vi "Populate Valid Y Variable Pointer IDs.vi"(8 "error in (no error)":errorcluster, 11 "Conditional Dialog in":refnum<class "Conditional Dialog.lvclass">) -> (0 "error out":errorcluster, 3 "Conditional Dialog out":refnum<class "Conditional Dialog.lvclass">)   [LabVIEW 2017, in "Conditional Dialog.lvclass"]
uses:
  <vilib>/gpm_packages/@cs/Test-executive-builder/Source/Test Executive Builder Dialogs/Edit Conditional Dialog/Conditional Dialog.lvclass
  <vilib>/gpm_packages/@cs/Test-executive-builder/Source/Test Executive Builder Dialogs/Edit Conditional Dialog/Conditional Dialog.lvclass/Conditional Dialog.ctl
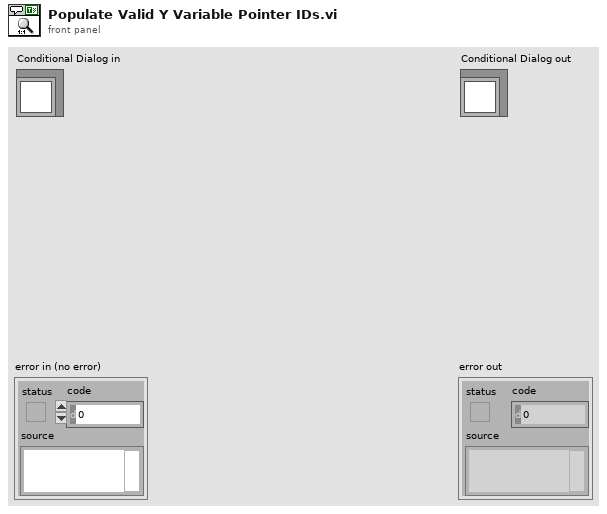
[diagram p1: front panel]
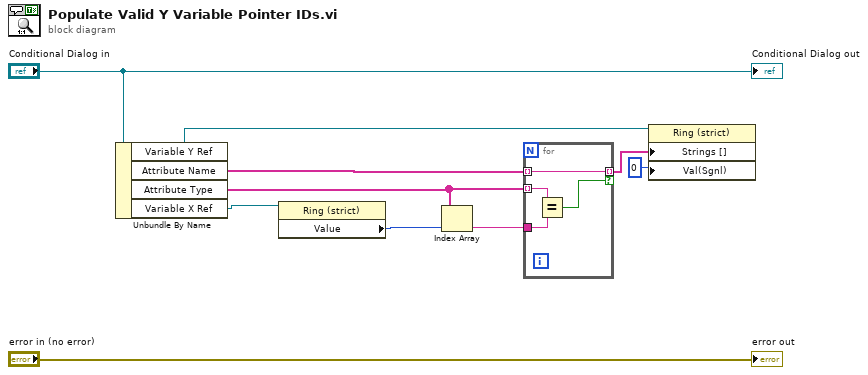
[diagram p0: block diagram]
diagram:
  n1 = Unbundle By Name("Conditional Dialog in") -> ("Variable Y Ref"=w3:refnum<vi>, "Attribute Name"=w4:string[], "Attribute Type"=w6:string[], "Variable X Ref"=w8:refnum<vi>)
  n2 = property class="Ring (strict)"(reference=w8) -> ("Value"=w7:u16)  [unwired: 1 in, 2 out]
  n3 = Index Array(array=w6, index=w7) -> (element=w5:string)
  n4 = for {
    tunnel: w6 -> [w13] mode=indexing
    tunnel: w5 -> [w14]
    tunnel: w4 -> [w12] mode=indexing
    tunnel: [w12] -> w2 mode=indexing if=w11
    n5 = Equal?(x=w13, y=w14) -> (x = y?=w11:bool)
  }
  n6 = property class="Ring (strict)"(reference=w3, "Strings []"=w2, "Val(Sgnl)"=u16 0 ("Value (Signaling)")) -> ()  [unwired: 1 in, 2 out]
  "error out" <- "error in (no error)"
  "Conditional Dialog out" <- "Conditional Dialog in"
